vi "Start Measurement.vi"(8 "error in (no error)":errorcluster, 10 "Launch Measurements Message in":refnum<class "Launch Measurements Message.lvclass">, 11 "Controller in":refnum<class "Controller.lvclass">) -> (0 "error out":errorcluster, 3 "Controller out":refnum<class "Controller.lvclass">)   [LabVIEW 2017, in "Controller Actor.lvlib" / "Controller.lvclass"]
uses:
  Controller.lvclass
  C:/Program Files (x86)/National Instruments/LabVIEW 2017/vi.lib/ActorFramework/Actor/Actor.lvclass
  Messages/Launch Measurements Message/Launch Measurements Message.lvclass
  Messages/Launch Measurements Message/Launch Measurements Message.lvclass/Launch Measurements Message.ctl
  Measurement Actor/Iteration Count.ctl
  Measurement Actor/Measurement.lvclass/Measurement.ctl
  <vilib>/ActorFramework/Actor/Actor.lvclass/Actor.ctl
  <vilib>/ActorFramework/Message Enqueuer/Message Enqueuer.lvclass/Message Enqueuer.ctl
  Measurement Actor/Accessors/Write Time Measurement Requested.vi
  Measurement Actor/Write GUID.vi
  Measurement Actor/Accessors/Write Continuous Run.vi
  Measurement Actor/Accessors/Read Step Configuration.vi
  Messages/Launch Measurements Message/Read Measurement Name.vi
  Messages/Launch Measurements Message/Read Device Names.vi
  Messages/Launch Measurements Message/Read Show FP_.vi
  Messages/Launch Measurements Message/Read Time Measurement Requested 2.vi
  Messages/Launch Measurements Message/Read GUID.vi
  Messages/Launch Measurements Message/Read Continuous Run 2.vi
  Messages/Launch Measurements Message/Read Iterations.vi
  <vilib>/ActorFramework/Message Enqueuer/Init from Existing Queue.vi
  Measurement Actor/Measurement.lvclass
  Measurement Actor/Properties/Write Array of Hardware 2.vi
  Measurement Actor/Properties/Write Show UI While Running 2.vi
  Measurement Actor/Configuration/Step Configuration.lvclass
  <vilib>/ActorFramework/Message Enqueuer/Message Enqueuer.lvclass
  <vilib>/ActorFramework/Actor/Actor.lvclass
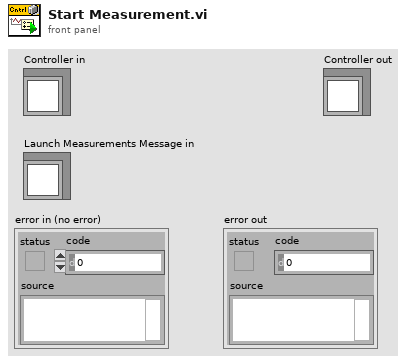
[diagram p1: front panel]
types:
  T1 = typedef "Measurement Actor.lvlib/Measurement.lvclass/Iteration Count.ctl" = cluster{"Desired Iterations":i32, "Current":i32}
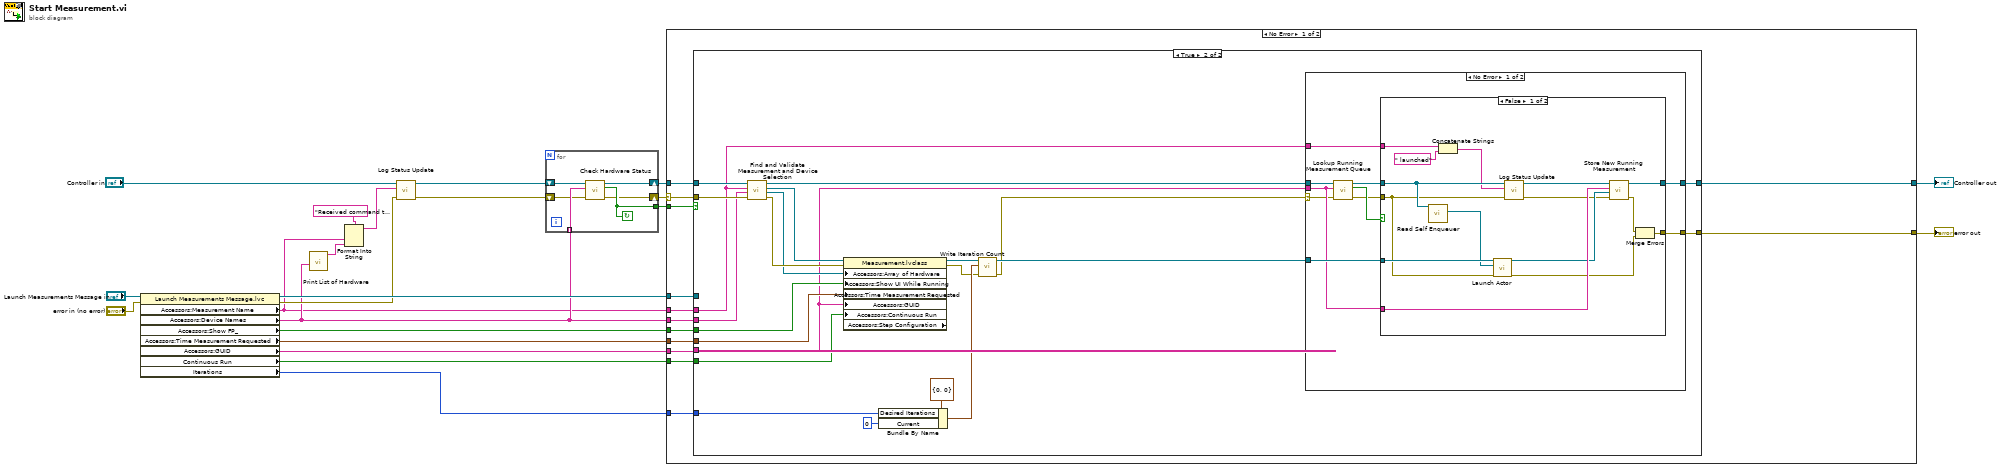
[diagram p0: block diagram]
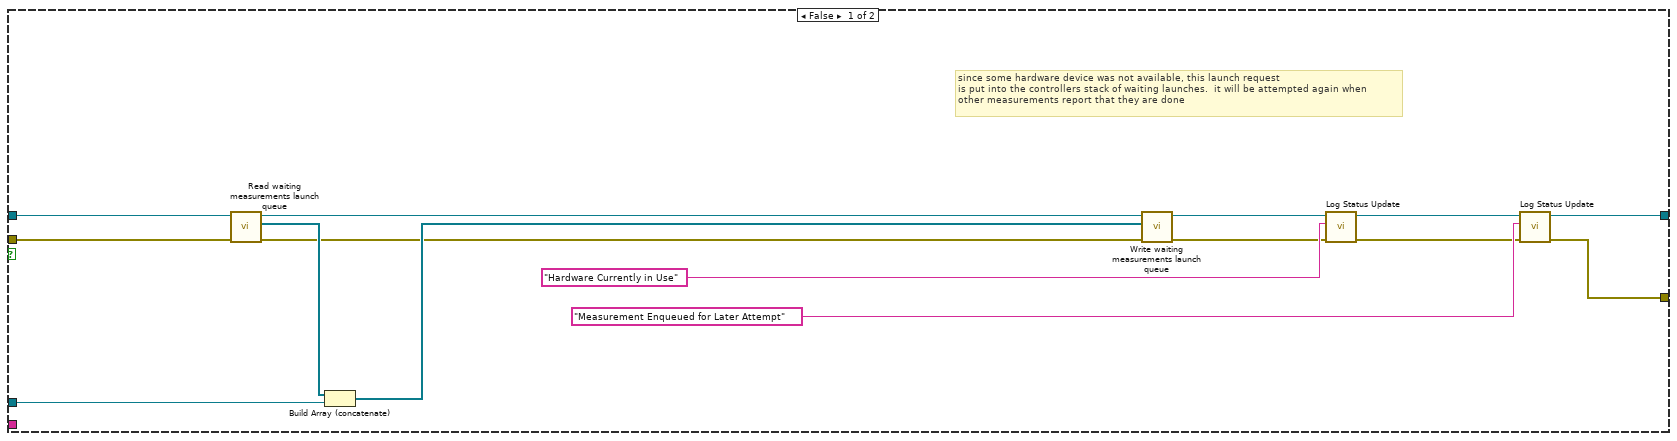
[diagram p2: hidden frame]
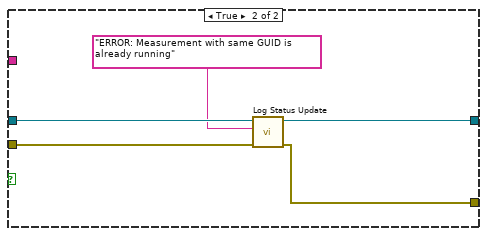
[diagram p3: hidden frame]
diagram:
  n1 = property class="Launch Measurements Message.lvc"(reference="Launch Measurements Message in", error in="error in (no error)") -> (reference out=w12:refnum<class "Launch Measurements Message.lvclass">, error out=w7:errorcluster, "Accessors:Measurement Name"=w3:string, "Accessors:Device Names"=w6:string[], "Accessors:Show FP_"=w9:bool, "Accessors:Time Measurement Requested"=w8:timestamp, "Accessors:GUID"=w11:string, "Continuous Run"=w2:bool, "Iterations"=w1:i32)
  n2 = call "Print List of Hardware.vi"("Device Names"=w6) -> ("String"=w21:string)  [unwired: 10 in]
  n3 = Format Into String(format string="Received command to run %s using %s", w3, w21) -> (resulting string=w20:string)  [unwired: 2 in, 1 out]
  n4 = call-dynamic "Log Status Update.vi"("error in (no error)"=w7, "String"=w20, "Controller in"="Controller in") -> ("error out"=w4:errorcluster, "Controller out"=w5:refnum<class "Controller.lvclass">)  [unwired: 7 in]
  n5 = for {
    shift-right: [w27] -> w17
    shift-left: w5 -> [w28]
    tunnel: w6 -> [w26] mode=indexing
    tunnel: [w25] -> w18
    shift-right: [w24] -> w16
    shift-left: w4 -> [w23]
    stop <- w25 continue-if-true
    n6 = call "Check Hardware Status.vi"("error in (no error)"=w23, "Device Name"=w26, "Controller in"=w28) -> ("error out"=w24:errorcluster, "Available?"=w25:bool, "Controller out"=w27:refnum<class "Controller.lvclass">)  [unwired: 6 in]
  }
  n7 = case shown="No Error" w16 {
    selector: w16 -> [w32 w112]
    tunnel: w18 -> [w41 _]
    tunnel: w17 -> [w33 w111]
    tunnel: [w40 w111] -> w14
    tunnel: w11 -> [w39 _]
    tunnel: [w38 w112] -> w13
    tunnel: w12 -> [w37 _]
    tunnel: w9 -> [w36 _]
    tunnel: w8 -> [w35 _]
    tunnel: w3 -> [w34 _]
    tunnel: w6 -> [w31 _]
    tunnel: w2 -> [w30 _]
    tunnel: w1 -> [w29 _]
    frame No Error {
      n8 = case shown="True" w41 {
        tunnel: [w43 w78] -> w40
        tunnel: w33 -> [w54 w77]
        tunnel: w32 -> [w52 w76]
        tunnel: [w44 w75] -> w38
        tunnel: w39 -> [_ w57]
        tunnel: w37 -> [w42 _]
        tunnel: w36 -> [_ w67]
        tunnel: w35 -> [_ w68]
        tunnel: w34 -> [_ w69]
        tunnel: w31 -> [_ w70]
        tunnel: w30 -> [_ w66]
        tunnel: w29 -> [_ w61]
        frame False {
          # "since some hardware device was not available, this launch request\nis put into the controllers stack of waiting launches.  it will be attempted again when\nother measurements report that they are done"
          n9 = call "Read waiting measurements launch queue.vi"("error in (no error)"=w52, "Controller in"=w54) -> ("error out"=w51:errorcluster, "stack of waiting msmt requests"=w56:refnum<class "Launch Measurements Message.lvclass">[], "Controller out"=w55:refnum<class "Controller.lvclass">)  [unwired: 7 in]
          n10 = Build Array (concatenate)(w56, w42) -> (w53:refnum<class "Launch Measurements Message.lvclass">[])
          n11 = call "Write waiting measurements launch queue.vi"("error in (no error)"=w51, "stack of waiting msmt requests"=w53, "Controller in"=w55) -> ("error out"=w46:errorcluster, "Controller out"=w47:refnum<class "Controller.lvclass">)  [unwired: 7 in]
          n12 = call-dynamic "Log Status Update.vi"("error in (no error)"=w46, "String"="Hardware Currently in Use", "Controller in"=w47) -> ("error out"=w45:errorcluster, "Controller out"=w48:refnum<class "Controller.lvclass">)  [unwired: 7 in]
          n13 = call-dynamic "Log Status Update.vi"("error in (no error)"=w45, "String"="Measurement Enqueued for Later Attempt", "Controller in"=w48) -> ("error out"=w44:errorcluster, "Controller out"=w43:refnum<class "Controller.lvclass">)  [unwired: 7 in]
        }
        frame True {
          n14 = call "Find and Validate Measurement and Device Selection.vi"("error in (no error)"=w76, "Device Names"=w70, "Measurement Name"=w69, "Controller in"=w77) -> ("error out"=w73:errorcluster, "Hardware Objects"=w72:refnum<class "Hardware.lvclass">[], "Measurement out"=w71:refnum<class "Measurement.lvclass">, "Controller out"=w74:refnum<class "Controller.lvclass">)  [unwired: 4 in]
          n15 = property class="Measurement.lvclass" props=["Accessors:Array of Hardware", "Accessors:Show UI While Running", "Accessors:Time Measurement Requested", "Accessors:GUID", "Accessors:Continuous Run", "Accessors:Step Configuration"](reference=w71, error in=w73, "Accessors:Array of Hardware"=w72, "Accessors:Show UI While Running"=w67, "Accessors:Time Measurement Requested"=w68, "Accessors:GUID"=w57, "Accessors:Continuous Run"=w66) -> (reference out=w65:refnum<class "Measurement.lvclass">, error out=w60:errorcluster)  [unwired: 1 out]
          n16 = Bundle By Name(cluster=T1 {"Desired Iterations"=0, "Current"=0} ("Iteration Count"), "Desired Iterations"=w61, "Current"=0) -> (w62:T1)
          n17 = call "Write Iteration Count.vi"("error in (no error)"=w60, "Iteration Count"=w62, "Measurement in"=w65) -> ("error out"=w58:errorcluster, "Measurement out"=w64:refnum<class "Measurement.lvclass">)  [unwired: 7 in]
          n18 = case shown="No Error" w58 {
            selector: w58 -> [w80 w110]
            tunnel: [w88 w109] -> w78
            tunnel: w64 -> [w84 _]
            tunnel: w74 -> [w83 w109]
            tunnel: w57 -> [w82 _]
            tunnel: [w81 w110] -> w75
            tunnel: w69 -> [w79 _]
            frame No Error {
              n19 = call "Lookup Running Measurement Queue.vi"("error in (no error)"=w80, "Measurement Name.Harware()"=w82, "Controller in"=w83) -> ("error out"=w85:errorcluster, "Found?"=w86:bool, "Controller out"=w87:refnum<class "Controller.lvclass">)  [unwired: 5 in, 1 out]
              n20 = case shown="False" w86 {
                tunnel: [w103 w107] -> w88
                tunnel: w84 -> [w102 _]
                tunnel: w82 -> [w101 _]
                tunnel: w87 -> [w99 w108]
                tunnel: w85 -> [w93 w105]
                tunnel: [w90 w104] -> w81
                tunnel: w79 -> [w89 _]
                frame False {
                  n21 = call <vilib>:"Read Self Enqueuer.vi"("Actor"=w99) -> ("Self Enqueuer"=w98:refnum<class "Message Enqueuer.lvclass">)  [unwired: 10 in]
                  n22 = Concatenate Strings(w89, " launched" ("string")) -> (w95:string)
                  n23 = call <vilib>:"Launch Actor.vi"("error in (no error)"=w93, "Actor-to-Caller Enqueuer"=w98, "Actor"=w102) -> ("error out"=w91:errorcluster, "Caller-To-Actor Enqueuer"=w97:refnum<class "Message Enqueuer.lvclass">)  [unwired: 7 in]
                  n24 = call-dynamic "Log Status Update.vi"("error in (no error)"=w93, "String"=w95, "Controller in"=w99) -> ("error out"=w94:errorcluster, "Controller out"=w96:refnum<class "Controller.lvclass">)  [unwired: 7 in]
                  n25 = call "Store New Running Measurement.vi"("error in (no error)"=w94, "Caller-To-Actor Enqueuer"=w97, "name"=w101, "Controller in"=w96) -> ("error out"=w92:errorcluster, "Controller out"=w103:refnum<class "Controller.lvclass">)  [unwired: 6 in]
                  n26 = Merge Errors(w92, w91) -> (w90:errorcluster)
                }
                frame True {
                  n27 = call-dynamic "Log Status Update.vi"("error in (no error)"=w105, "String"="ERROR: Measurement with same GUID is already running", "Controller in"=w108) -> ("error out"=w104:errorcluster, "Controller out"=w107:refnum<class "Controller.lvclass">)  [unwired: 7 in]
                }
              }
            }
            frame Error {
            }
          }
        }
      }
    }
    frame Error {
    }
  }
  "error out" <- w13
  "Controller out" <- w14
